vi "Write Parent State.vi"(8 "error in (no error)":errorcluster, 10 "State.lvlib:State.lvclass":refnum<class "State.lvclass">, 11 "Container State in":refnum<class "Container State.lvclass">) -> (0 "error out":errorcluster, 3 "Container State out":refnum<class "Container State.lvclass">)   [LabVIEW 2024, in "State.lvlib" / "Container State.lvclass"]
uses:
  Container State.lvclass
  Container State.lvclass/Container State.ctl
  State/State.lvclass
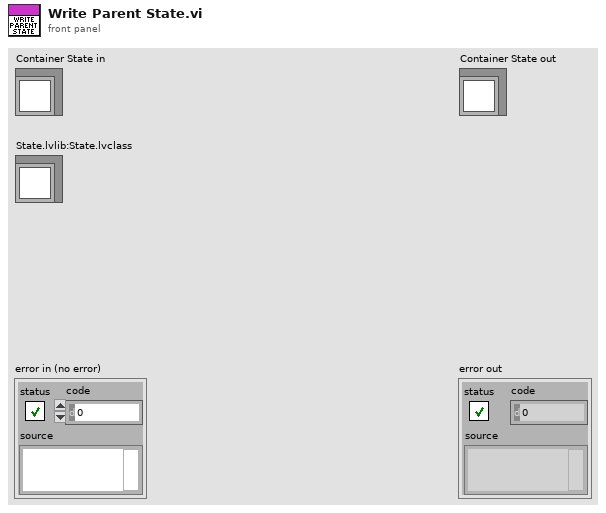
[diagram p1: front panel]
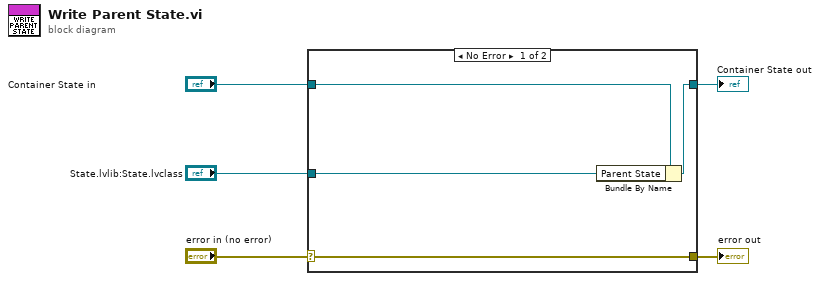
[diagram p0: block diagram]
diagram:
  n1 = case shown="No Error" "error in (no error)" {
    selector: "error in (no error)" -> [w9 w10]
    tunnel: [w9 w10] -> w4
    tunnel: [w7 w11] -> w2
    tunnel: "Container State in" -> [w8 w11]
    tunnel: "State.lvlib:State.lvclass" -> [w6 _]
    frame No Error {
      n2 = Bundle By Name(cluster=w8, "Parent State"=w6) -> (w7:refnum<class "Container State.lvclass">)
    }
    frame Error {
    }
  }
  "error out" <- w4
  "Container State out" <- w2
